vi "Filter Meta.vi"(8 "error in (no error)":errorcluster, 9 "Meta":T1[](array[typedef]), 10 "Elements":refnum<class "Config Element.lvclass">[](array[class]), 11 "Config Manager in":refnum<class "Config Manager.lvclass">) -> (0 "error out":errorcluster, 2 "Matches":refnum<class "Config Element.lvclass">[](array[class]), 3 "Config Manager out":refnum<class "Config Manager.lvclass">)   [LabVIEW 2020, in "CDM-Config.lvlib" / "Config Manager.lvclass"]
uses:
  Config Manager.lvclass
  Config Element/Config Element.lvclass
  Meta Data.ctl
  b47f34b2-d53d-48ea-85ed-16fae7f57de2.vi
  <vilib>/Comparison/Equal/Equal Functor/Equal Functor.lvclass
  CDM-Config.lvlib
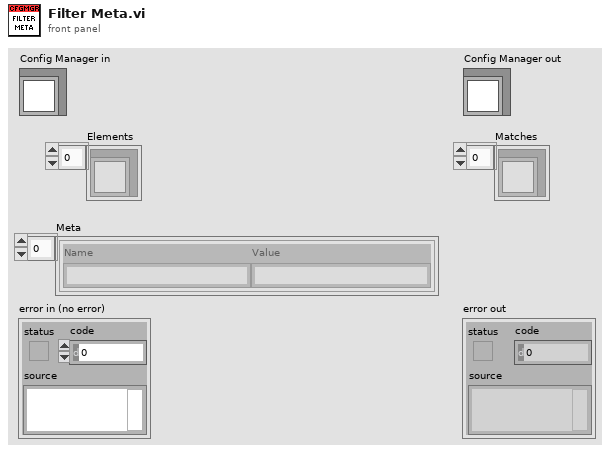
[diagram p1: front panel]
types:
  T1 = typedef "CDM-Config.lvlib/Meta Data.ctl" = cluster{"Name":string, "Value":string}
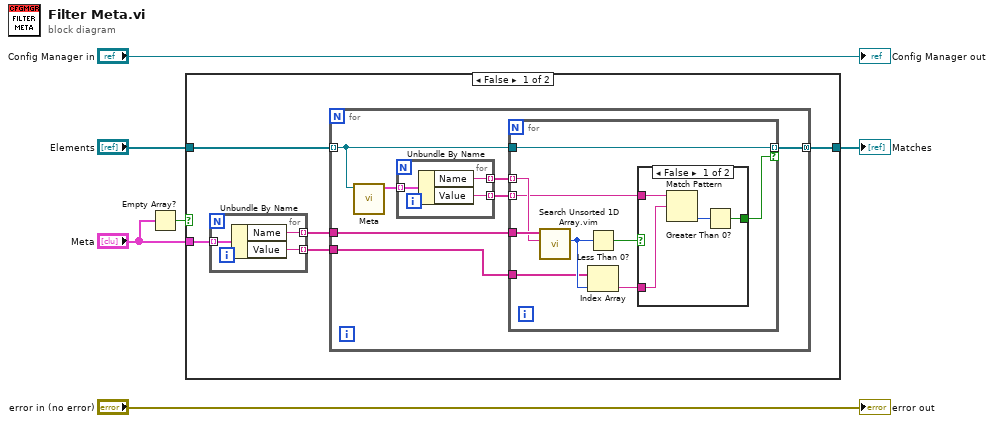
[diagram p0: block diagram]
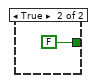
[diagram p2: hidden frame]
diagram:
  n1 = Empty Array?(array="Meta") -> (empty?=w1:bool)
  n2 = case shown="False" w1 {
    tunnel: "Elements" -> [w11 w39]
    tunnel: [w8 w39] -> w3
    tunnel: "Meta" -> [w7 _]
    frame False {
      n3 = for {
        tunnel: w7 -> [w38] mode=indexing
        tunnel: [w37] -> w10 mode=indexing
        tunnel: [w36] -> w9 mode=indexing
        n4 = Unbundle By Name(w38) -> ("Name"=w37:string, "Value"=w36:string)
      }
      n5 = for {
        tunnel: w11 -> [w14] mode=indexing
        tunnel: w10 -> [w17]
        tunnel: w9 -> [w13]
        tunnel: [w12] -> w8 mode=concatenating
        n6 = call "Meta.vi"("Config Element in"=w14) -> ("Meta Data"=w18:T1[])  [unwired: 9 in, 1 out]
        n7 = for {
          tunnel: w18 -> [w35] mode=indexing
          tunnel: [w34] -> w16 mode=indexing
          tunnel: [w33] -> w15 mode=indexing
          n8 = Unbundle By Name(w35) -> ("Name"=w34:string, "Value"=w33:string)
        }
        n9 = for {
          tunnel: w17 -> [w26]
          tunnel: w16 -> [w25] mode=indexing
          tunnel: w15 -> [w21] mode=indexing
          tunnel: w14 -> [w20]
          tunnel: w13 -> [w24]
          tunnel: [w20] -> w12 mode=indexing if=w19
          n10 = call "Search Unsorted 1D Array.vim"("element"=w25, "unsorted 1D array"=w26) -> ("index of element"=w27:i32)  [unwired: 9 in]
          n11 = Less Than 0?(x=w27) -> (x < 0?=w23:bool)
          n12 = Index Array(array=w24, index=w27) -> (element=w22:string)
          n13 = case shown="False" w23 {
            tunnel: w22 -> [w30 _]
            tunnel: w21 -> [w31 _]
            tunnel: [w28 FALSE] -> w19
            frame False {
              n14 = Match Pattern(string=w31, regular expression=w30) -> (offset past match=w29:i32)  [unwired: 1 in, 3 out]
              n15 = Greater Than 0?(x=w29) -> (x > 0?=w28:bool)
            }
            frame True {
            }
          }
        }
      }
    }
    frame True {
    }
  }
  "Matches" <- w3
  "error out" <- "error in (no error)"
  "Config Manager out" <- "Config Manager in"
